vi "FlatToRichcalculator_AddResponse.vi"(5 "OutputClusterType":T1, 11 "InputCluster":T2) -> (3 "OutputCluster":T1)   [LabVIEW 2025, in "calculator_client.lvlib"]
uses:
  calculator_client.lvlib
  calculator_AddResponse_Flat.ctl
  calculator_AddResponse.ctl
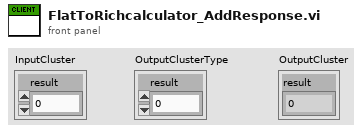
[diagram p1: front panel]
types:
  T1 = typedef "calculator_client.lvlib/calculator_AddResponse.ctl" = cluster{"result":dbl}
  T2 = typedef "calculator_client.lvlib/calculator_AddResponse_Flat.ctl" = cluster{"result":dbl}
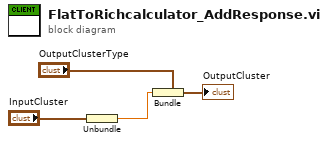
[diagram p0: block diagram]
diagram:
  n1 = Unbundle "Unbundle"("InputCluster") -> ("result"=w1:dbl)
  n2 = Bundle "Bundle"(cluster="OutputClusterType", "result"=w1) -> (→"OutputCluster":T1)
